vi "Get settings chain.vi"(8 "error in (no error)":errorcluster, 11 "wavefront sensorBase in":refnum<class "wavefront sensor.lvclass">) -> (0 "error out":errorcluster, 1 "class name":string[](array[string]), 2 "settings":variant[](array[variant]), 3 "wavefront sensorBase out":refnum<class "wavefront sensor.lvclass">)   [LabVIEW 2012, in "wavefront sensor.lvclass"]
doc: "Returns an array of variants containing the settings clusters of each class in the inheritance chain (lowest child class first), together with an array of all class names in the inheritance chain.\n\nFor classes without settings cluster, the settings chain contains empty variants."
uses:
  wavefront sensor.lvclass
  <vilib>/Distrio/Murmex/Murmex/Murmex.lvclass
  wavefront sensor.lvclass/wavefront sensor.ctl
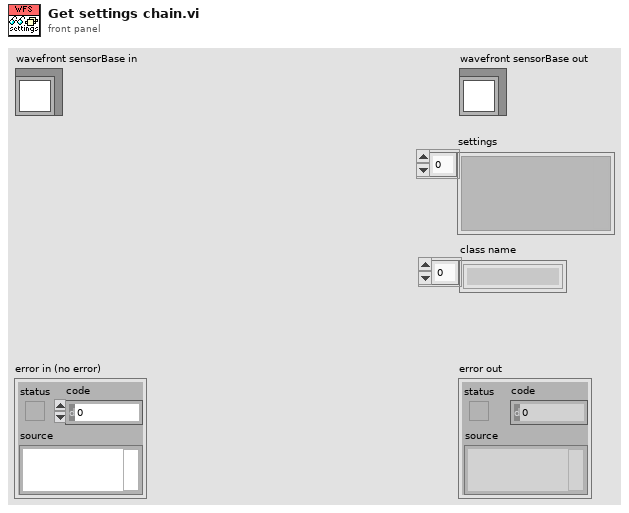
[diagram p1: front panel]
types:
  T1 = typedef "wavefront sensor.lvclass/settings.ctl" = cluster{"Numeric":dbl}
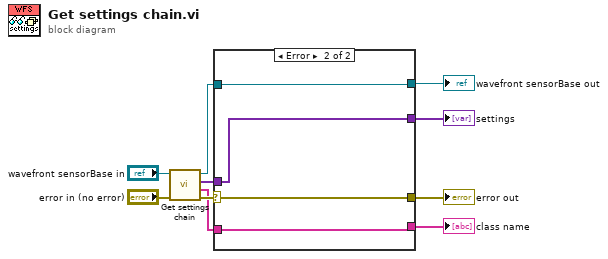
[diagram p0: block diagram]
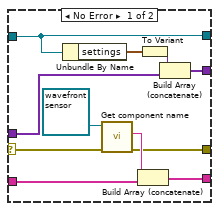
[diagram p2: hidden frame]
diagram:
  n1 = call-parent "Get settings chain.vi"("error in (no error)"="error in (no error)", "MurmexBase in"="wavefront sensorBase in") -> ("error out"=w8:errorcluster, "class name"=w1:string[], "settings"=w3:variant[], "MurmexBase out"=w6:refnum<class "wavefront sensor.lvclass">)  [unwired: 6 in]
  n2 = case shown="Error" w8 {
    selector: w8 -> [w18 w24]
    tunnel: [w17 w24] -> w7
    tunnel: w6 -> [w15 w25]
    tunnel: [w15 w25] -> w5
    tunnel: [w14 w23] -> w4
    tunnel: w3 -> [w13 w23]
    tunnel: [w12 w22] -> w2
    tunnel: w1 -> [w11 w22]
    frame No Error {
      n3 = Unbundle By Name(w15) -> ("settings"=w21:T1)
      n4 = call <vilib>:"Get component name.vi"("error in (no error)"=w18, "Murmex in"=refnum<class "wavefront sensor.lvclass"> refnum ("wavefront sensor")) -> ("error out"=w17:errorcluster, "component name"=w19:string)  [unwired: 7 in, 1 out]
      n5 = Build Array (concatenate)(w19, w11) -> (w12:string[])
      n6 = To Variant(anything=w21) -> (Variant=w20:variant)
      n7 = Build Array (concatenate)(w20, w13) -> (w14:variant[])
    }
    frame Error {
    }
  }
  "error out" <- w7
  "wavefront sensorBase out" <- w5
  "settings" <- w4
  "class name" <- w2
